vi "Set Limits on Configure Device.vi"(8 "error in (no error)":errorcluster, 10 "Toggle8 controls cluster":T1, 11 "Toggle 8 in":refnum<class "Toggle 8.lvclass">) -> (0 "error out":errorcluster, 3 "Toggle 8 out":refnum<class "Toggle 8.lvclass">)   [LabVIEW 2020, in "Toggle 8.lvclass"]
uses:
  Toggle 8.lvclass
  C:/Sandbox/RF Bench/Source Code/WiSpry Test Framework/Devices/Device.lvclass
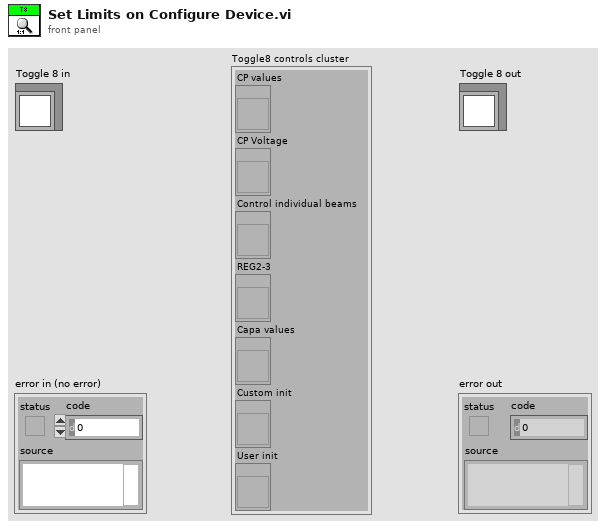
[diagram p1: front panel]
types:
  T1 = cluster{"CP values":refnum<vi>, "CP Voltage":refnum<vi>, "Control individual beams":refnum<vi>, "REG2-3":refnum<vi>, "Capa values":refnum<vi>, "Custom init":refnum<vi>, "User init":refnum<vi>}
  T2 = enum8{"Enabled", "Disabled", "Disabled and Grayed Out"}
  T3 = cluster{"Enable":bool, "User init values":string}
  T4 = typedef "Toggle 8.lvclass/Test Sequence.ctl" = cluster{"CP values":string, "Charge Pump values":enum16{"CP 24V", "CP 26V", "CP 28V", "CP 30V", "CP 31V", "CP 32V", "CP 33V", "CP 34V", "CP 35V", "CP 36V", "CP 37V", "CP 38V", "CP 39V", "CP 40V", "CP 41V", "CP 42V", "CP 43V", "CP 44V", "CP 45V", "CP 46V", "CP 47V", "CP 48V", "CP 49V", "CP 50V", "CP 51V", "CP 52V", "CP 53V", "CP 54V", "CP 56V", "CP 58V", "CP 60V", "CP 62V"}[], "Charge Pump":T5[], "Control individual beams":bool, "OTP/beam values":dbl[], "Capa settings":T5[], "OTP Values string":string}
  T5 = typedef "PIC-Device.lvclass/Register to Write.ctl" = cluster{"Register":u32, "Value":u32, "Dev Address":u32, "Physical Adress":u32}
  T6 = enum16{"CP 24V", "CP 26V", "CP 28V", "CP 30V", "CP 31V", "CP 32V", "CP 33V", "CP 34V", "CP 35V", "CP 36V", "CP 37V", "CP 38V", "CP 39V", "CP 40V", "CP 41V", "CP 42V", "CP 43V", "CP 44V", "CP 45V", "CP 46V", "CP 47V", "CP 48V", "CP 49V", "CP 50V", "CP 51V", "CP 52V", "CP 53V", "CP 54V", "CP 56V", "CP 58V", "CP 60V", "CP 62V"}[]
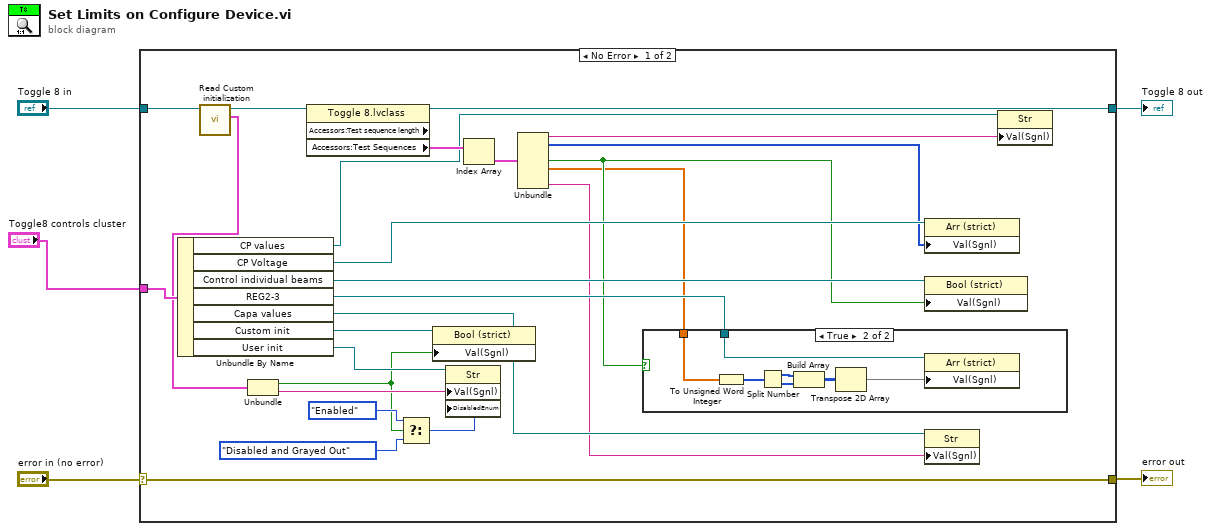
[diagram p0: block diagram]
diagram:
  n1 = case shown="No Error" "error in (no error)" {
    selector: "error in (no error)" -> [w30 w39]
    tunnel: [w30 w39] -> w4
    tunnel: [w22 w38] -> w2
    tunnel: "Toggle 8 in" -> [w13 w38]
    tunnel: "Toggle8 controls cluster" -> [w29 _]
    frame No Error {
      n2 = Unbundle By Name(w29) -> ("CP values"=w16:refnum<vi>, "CP Voltage"=w28:refnum<vi>, "Control individual beams"=w25:refnum<vi>, "REG2-3"=w26:refnum<vi>, "Capa values"=w27:refnum<vi>, "Custom init"=w15:refnum<vi>, "User init"=w14:refnum<vi>)
      n3 = call-dynamic "Read Custom initialization.vi"("Toggle 8 in"=w13) -> ("Custom initialization"=w8:T3, "Toggle 8 out"=w12:refnum<class "Toggle 8.lvclass">)  [unwired: 9 in]
      n4 = Unbundle(w8) -> ("Enable"=w6:bool, "User init values"=w7:string)
      n5 = property class="Toggle 8.lvclass" props=["Accessors:Test sequence length", "Accessors:Test Sequences"](reference=w12) -> (reference out=w22:refnum<class "Toggle 8.lvclass">, "Accessors:Test Sequences"=w24:T4[])  [unwired: 1 in, 2 out]
      n6 = Select(t=T2."Enabled" ("Disabled"), s=w6, f=T2."Disabled and Grayed Out" ("Disabled")) -> (s? t:f=w9:T2)
      n7 = property class="Bool (strict)"(reference=w15, "Val(Sgnl)"=w6) -> ()  [unwired: 1 in, 2 out]
      n8 = property class="Str"(reference=w14, "Val(Sgnl)"=w7, "DisabledEnum"=w9) -> ()  [unwired: 1 in, 2 out]
      n9 = Index Array(array=w24) -> (element=w23:T4)  [unwired: 1 in]
      n10 = Unbundle(w23) -> ("CP values"=w17:string, "Charge Pump values"=w20:T6, "Control individual beams"=w19:bool, "OTP/beam values"=w18:dbl[], "OTP Values string"=w21:string)  [unwired: 2 out]
      n11 = case shown="True" w19 {
        tunnel: w26 -> [_ w37]
        tunnel: w18 -> [_ w33]
        frame False {
        }
        frame True {
          n12 = To Unsigned Word Integer(number=w33) -> (unsigned 16bit integer=w32:u16[])
          n13 = Split Number(x=w32) -> (hi(x)=w36:u8[], lo(x)=w35:u8[])
          n14 = Build Array(w36, w35) -> (w34:u8[][])
          n15 = Transpose 2D Array(2D array=w34) -> (transposed array=w31:u8[][])
          n16 = property class="Arr (strict)"(reference=w37, "Val(Sgnl)"=w31) -> ()  [unwired: 1 in, 2 out]
        }
      }
      n17 = property class="Arr (strict)"(reference=w28, "Val(Sgnl)"=w20) -> ()  [unwired: 1 in, 2 out]
      n18 = property class="Bool (strict)"(reference=w25, "Val(Sgnl)"=w19) -> ()  [unwired: 1 in, 2 out]
      n19 = property class="Str"(reference=w27, "Val(Sgnl)"=w21) -> ()  [unwired: 1 in, 2 out]
      n20 = property class="Str"(reference=w16, "Val(Sgnl)"=w17) -> ()  [unwired: 1 in, 2 out]
    }
    frame Error {
    }
  }
  "error out" <- w4
  "Toggle 8 out" <- w2
